vi "Kinect - Weak detect (SubVI).vi"(7 "error in (no error)":errorcluster, 10 "Array of Joint Positions In":dbl[][](array[numeric])) -> (0 "error out":errorcluster, 2 "Boolean":bool, 3 "Array of Joint Positions Out":dbl[][](array[numeric]))   [LabVIEW 2014]
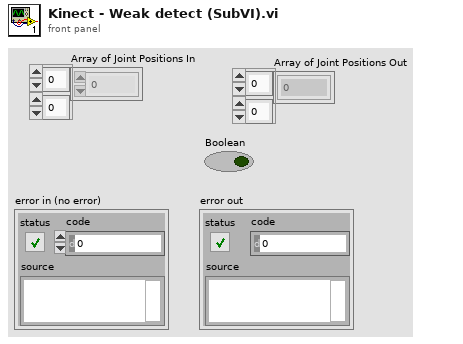
[diagram p1: front panel]
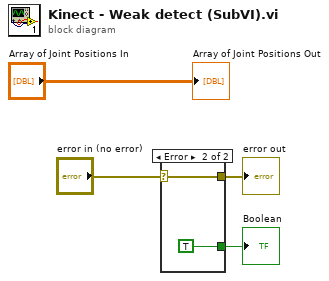
[diagram p0: block diagram]
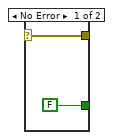
[diagram p2: hidden frame]
diagram:
  n1 = case shown="Error" "error in (no error)" {
    selector: "error in (no error)" -> [w6 w7]
    tunnel: [FALSE TRUE] -> w3
    tunnel: [w6 w7] -> w4
    frame No Error {
    }
    frame Error {
    }
  }
  "error out" <- w4
  "Boolean" <- w3
  "Array of Joint Positions Out" <- "Array of Joint Positions In"
